vi "OAT Demodulation with Decimation (N Freq, 1 Ch).vi"(0 "x[n]":dbl[](array[numeric]) format="%.2f", 1 "reset? (True)":bool=TRUE, 2 "zero delay? (F)":bool, 5 "fs":dbl=1.0 format="%.2f", 9 "fc [Hz]":dbl[](array[numeric])=[0.0] format="%.2f", 11 "decimation factor":i32=16, 12 "stop band attenuation":u16(ring) items=["72 dB", "96 dB", "120 dB"], 14 "phase setting":T1) -> (3 "lags":i32, 4 "magnitudes (RMS)":dbl[][](array[numeric]) format="%.2f", 6 "phase lag":dbl[][](array[numeric]) format="%.2f", 10 "new fs [Hz]":dbl format="%.2f", 15 "error out":errorcluster)   [LabVIEW 2017, in "SoundVib_Resampling.lvlib"]
uses:
  <vilib>/addons/Sound and Vibration/Order Analysis/Resample Order Tracking/SoundVib_Resampling.lvlib
  <vilib>/addons/Sound and Vibration/Order Analysis/Misc/OAT Convert Phase (1 channel).vi
  <vilib>/Analysis/NI_AALPro.lvlib
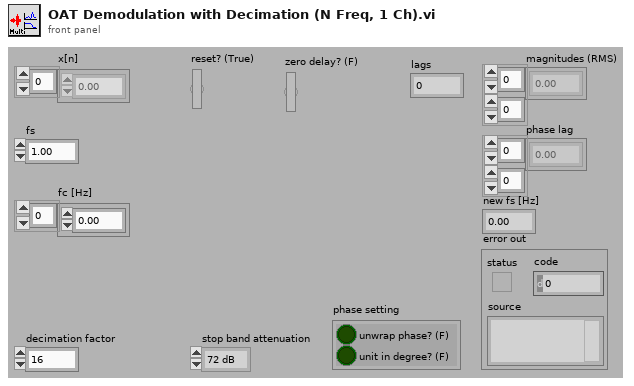
[diagram p1: front panel]
types:
  T1 = cluster{"unwrap phase? (F)":bool, "unit in degree? (F)":bool}
  T2 = typedef "OAT Decimation Filter.ctl" = cluster{"coefficients":dbl[], "factor":i32}
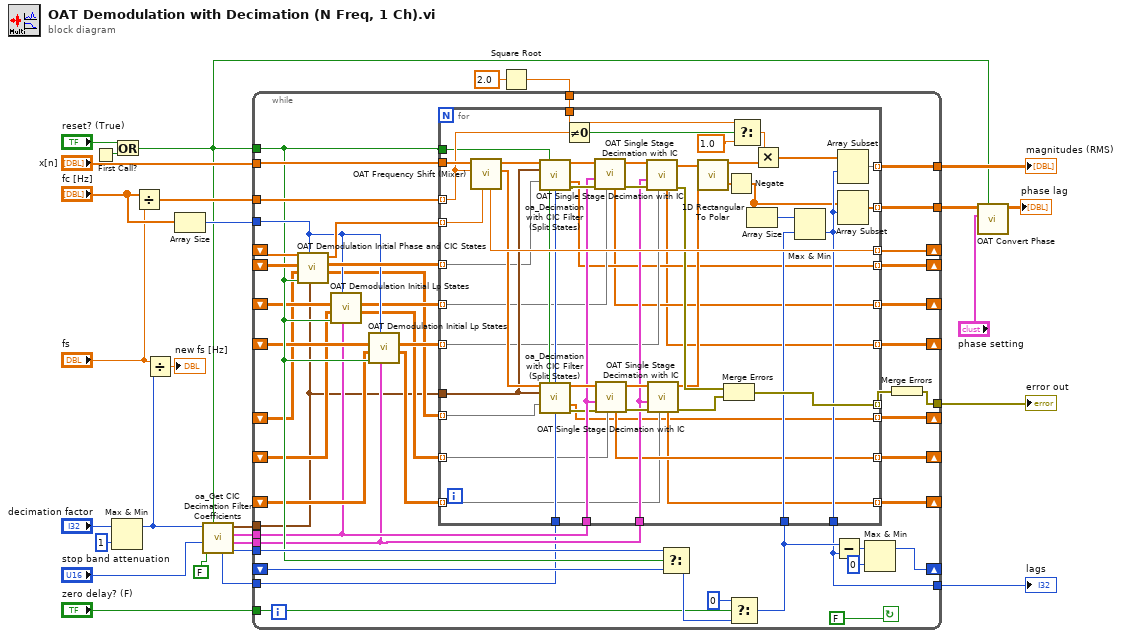
[diagram p0: block diagram]
diagram:
  n1 = First Call?() -> (First Call?: T/F=w17:bool)
  n2 = Max & Min(x="decimation factor", y=1) -> (max(x,y)=w8:i32)  [unwired: 1 out]
  n3 = Or(x="reset? (True)", y=w17) -> (x .or. y?=w10:bool)
  n4 = Divide(x="fc [Hz]", y="fs") -> (x/y=w28:dbl[])
  n5 = Divide(x="fs", y=w8) -> (x/y=→"new fs [Hz]":dbl)
  n6 = Array Size(array="fc [Hz]") -> (size(s)=w27:i32)
  n7 = call <vilib>:"oa_Get CIC Decimation Filter Coefficients.vi"("reset? (True)"=w10, "alias protect in final transition"=FALSE, "stop band attenuation"="stop band attenuation", "decimation/interpolation factor"=w8) -> ("delay"=w4:i32, "lp filter settings"=w1:T2, "compensation filter settings"=w2:T2, "CIC Settings"=w9:cluster{"Numeric":i32, i32, i32}, "interpolation factor"=w5:i32)  [unwired: 3 in]
  n8 = Square Root(x=2.0) -> (sqrt(x)=w25:dbl)
  n9 = while {
    tunnel: w25 -> [w29]
    tunnel: w27 -> [w50]
    shift-left: _ -> [w58]
    shift-right: [w56] -> _
    tunnel: w10 -> [w49]
    shift-left: _ -> [w57]
    shift-right: [w55] -> _
    shift-left: _ -> [w39]
    shift-right: [w46] -> _
    tunnel: w28 -> [w60]
    tunnel: "x[n]" -> [w61]
    tunnel: [w62] -> w13
    tunnel: [w63] -> w24
    tunnel: [w72] -> w15
    tunnel: [w30] -> w14
    shift-right: [w68] -> _
    shift-left: _ -> [w71]
    tunnel: w9 -> [w33]
    tunnel: w5 -> [w32]
    tunnel: w4 -> [w67]
    tunnel: "zero delay? (F)" -> [w64]
    shift-right: [w54] -> _
    shift-left: _ -> [w44]
    shift-right: [w51] -> _
    shift-left: _ -> [w42]
    shift-right: [w48] -> _
    shift-left: _ -> [w41]
    shift-right: [w47] -> _
    shift-left: _ -> [w40]
    tunnel: w2 -> [w35]
    tunnel: w1 -> [w34]
    stop <- FALSE continue-if-true
    n10 = call <vilib>:"OAT Demodulation Initial Phase and CIC States.vi"("CIC filter settings"=w33, "num of orders"=w50, "reset? (True)"=w49, "CIC Image in"=w41, "CIC Real in"=w57, "start phase in"=w58) -> ("CIC Image"=w38:dbl[][], "CIC Real"=w53:dbl[][], "start phase out"=w59:dbl[])  [unwired: 3 in]
    n11 = call <vilib>:"OAT Demodulation Initial Lp States.vi"("filter"=w35, "num of orders"=w50, "reset? (True)"=w49, "Lp Image in"=w40, "Lp Real in"=w44) -> ("Lp Image"=w37:dbl[][], "Lp Real"=w45:dbl[][])  [unwired: 5 in]
    n12 = call <vilib>:"OAT Demodulation Initial Lp States.vi"("filter"=w34, "num of orders"=w50, "reset? (True)"=w49, "Lp Image in"=w39, "Lp Real in"=w42) -> ("Lp Image"=w36:dbl[][], "Lp Real"=w43:dbl[][])  [unwired: 5 in]
    n13 = Select(t=w67, s=w49, f=w71) -> (s? t:f=w65:i32)
    n14 = Select(t=0 ("delay"), s=w64, f=w65) -> (s? t:f=w31:i32)
    n15 = for {
      tunnel: w61 -> [w120]
      tunnel: w60 -> [w109] mode=indexing
      tunnel: [w122] -> w56 mode=indexing
      tunnel: w59 -> [w86] mode=indexing
      tunnel: w29 -> [w107]
      tunnel: [w113] -> w62 mode=indexing
      tunnel: [w114] -> w63 mode=indexing
      tunnel: [w116] -> w52 mode=indexing
      tunnel: w31 -> [w111]
      tunnel: [w110] -> w30
      tunnel: w49 -> [w104]
      tunnel: w33 -> [w102]
      tunnel: w32 -> [w101]
      tunnel: w35 -> [w93]
      tunnel: w34 -> [w87]
      tunnel: w53 -> [w85] mode=indexing
      tunnel: [w82] -> w55 mode=indexing
      tunnel: w45 -> [w84] mode=indexing
      tunnel: [w81] -> w54 mode=indexing
      tunnel: w43 -> [w83] mode=indexing
      tunnel: [w80] -> w51 mode=indexing
      tunnel: w38 -> [w79] mode=indexing
      tunnel: [w74] -> w48 mode=indexing
      tunnel: w37 -> [w78] mode=indexing
      tunnel: [w77] -> w47 mode=indexing
      tunnel: w36 -> [w76] mode=indexing
      tunnel: [w75] -> w46 mode=indexing
      n16 = call <vilib>:"OAT Frequency Shift (Mixer).vi"("initial phase"=w86, "fc"=w109, "X"=w120) -> ("imaginary"=w119:dbl[], "real"=w118:dbl[], "final phase"=w122:dbl)  [unwired: 6 in]
      n17 = call <vilib>:"oa_Decimation with CIC Filter (Split States).vi"("x[n]"=w118, "reset? (True)"=w104, "CIC decimation setting"=w102, "CIC state"=w85, "interpolation factor"=w101) -> ("x[n] out"=w100:dbl[], "final CIC state"=w82:dbl[], "error out"=w97:errorcluster)  [unwired: 8 in]
      n18 = call <vilib>:"oa_Decimation with CIC Filter (Split States).vi"("x[n]"=w119, "reset? (True)"=w104, "CIC decimation setting"=w102, "CIC state"=w79, "interpolation factor"=w101) -> ("x[n] out"=w94:dbl[], "final CIC state"=w74:dbl[], "error out"=w90:errorcluster)  [unwired: 8 in]
      n19 = Not Equal To 0?(x=w109) -> (x != 0?=w108:bool)
      n20 = call <vilib>:"OAT Single Stage Decimation with IC.vi"("initial state"=w84, "error in (no error)"=w97, "filter"=w93, "X"=w100) -> ("error out"=w96:errorcluster, "Y"=w98:dbl[], "final state"=w81:dbl[])  [unwired: 5 in]
      n21 = call <vilib>:"OAT Single Stage Decimation with IC.vi"("initial state"=w78, "error in (no error)"=w90, "filter"=w93, "X"=w94) -> ("error out"=w92:errorcluster, "Y"=w91:dbl[], "final state"=w77:dbl[])  [unwired: 5 in]
      n22 = call <vilib>:"OAT Single Stage Decimation with IC.vi"("initial state"=w83, "error in (no error)"=w96, "filter"=w87, "X"=w98) -> ("error out"=w95:errorcluster, "Y"=w99:dbl[], "final state"=w80:dbl[])  [unwired: 5 in]
      n23 = call <vilib>:"OAT Single Stage Decimation with IC.vi"("initial state"=w76, "error in (no error)"=w92, "filter"=w87, "X"=w91) -> ("error out"=w89:errorcluster, "Y"=w88:dbl[], "final state"=w75:dbl[])  [unwired: 5 in]
      n24 = call <vilib>:"1D Rectangular To Polar.vi"("X"=w99, "Y"=w88) -> ("Magnitude"=w121:dbl[], "Phase"=w117:dbl[])  [unwired: 1 out]
      n25 = Merge Errors(w95, w89) -> (w116:errorcluster)
      n26 = Negate(x=w117) -> (-x=w103:dbl[])
      n27 = Select(t=w107, s=w108, f=1.0) -> (s? t:f=w106:dbl)
      n28 = Array Size(array=w103) -> (size(s)=w112:i32)
      n29 = Multiply(x=w106, y=w121) -> (x*y=w115:dbl[])
      n30 = Max & Min(x=w112, y=w111) -> (min(x,y)=w110:i32)  [unwired: 1 out]
      n31 = Array Subset(array=w115, index=w110) -> (w114:dbl[])  [unwired: 1 in]
      n32 = Array Subset(array=w103, index=w110) -> (w113:dbl[])  [unwired: 1 in]
    }
    n33 = Subtract(x=w31, y=w30) -> (x-y=w70:i32)
    n34 = Max & Min(x=w70, y=0) -> (max(x,y)=w68:i32)  [unwired: 1 out]
    n35 = Merge Errors(w52) -> (w72:errorcluster)
  }
  "error out" <- w15
  "magnitudes (RMS)" <- w24
  "lags" <- w14
  n36 = call-poly <vilib>:"OAT Convert Phase.vi"("reset (TRUE)"=w10, "desired phase setting"="phase setting", "phase in (rad)"=w13) -> ("phase out"=→"phase lag":dbl[][])  [unwired: 8 in]
